vi "Cannon Auto.vi"(1 "Cannon Info In":T2) -> (0 "Cannon Info Out":T2)   [LabVIEW 2013]
uses:
  <vilib>/Rock Robotics/WPI/Solenoid/WPI_SolenoidValue.ctl
panel:
  # "Togle"
  # "Togle"
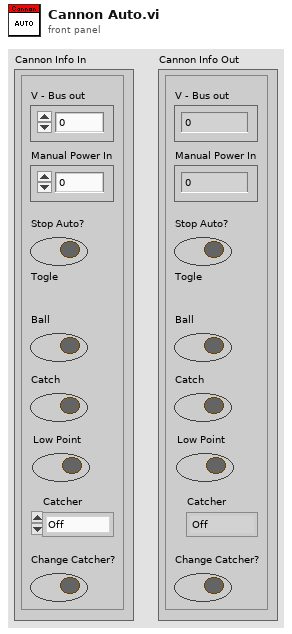
[diagram p1: front panel]
types:
  T1 = typedef "WPI_SolenoidValue.ctl" = enum16{"Off", "On", "Forward", "Reverse"}
  T2 = cluster{"V - Bus out":dbl, "Manual Power In":dbl, "Stop Auto?":bool, "Ball":bool, "Catch":bool, "Low Point":bool, "Catcher":T1, "Change Catcher?":bool}
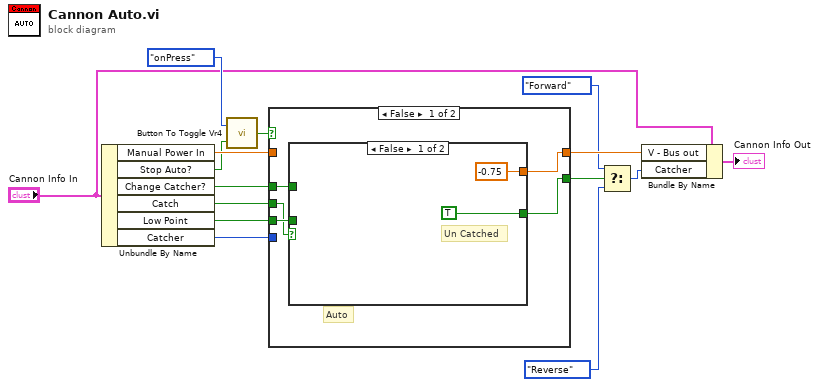
[diagram p0: block diagram]
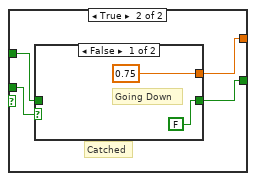
[diagram p2: hidden frame]
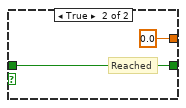
[diagram p3: hidden frame]
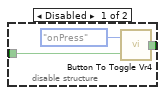
[diagram p5: hidden frame]
diagram:
  n1 = Unbundle By Name("Cannon Info In") -> ("Manual Power In"=w11:dbl, "Stop Auto?"=w1:bool, "Change Catcher?"=w3:bool, "Catch"=w13:bool, "Low Point"=w12:bool, "Catcher"=w2:T1)
  n2 = call "Button To Toggle Vr4.vi"("InValue"=w1, "Action"=enum16{"onPress", "onRelease", "Both"}."onPress") -> ("Result"=w14:bool)
  n3 = case shown="False" w14 {
    tunnel: w13 -> [w17 _]
    tunnel: w12 -> [w20 _]
    tunnel: w11 -> [_ w33]
    tunnel: w3 -> [w16 w32]
    tunnel: [w18 w33] -> w8
    tunnel: [w19 w31] -> w7
    tunnel: w2 -> [_ _]
    frame False {
      # "Auto"
      n4 = case shown="False" w17 {
        tunnel: w20 -> [_ w26]
        tunnel: [TRUE w24] -> w19
        tunnel: [-0.75 w25] -> w18
        tunnel: w16 -> [_ w23]
        frame False {
          # "Un Catched"
        }
        frame True {
          # "Catched"
          n5 = case shown="False" w26 {
            tunnel: [0.75 0.0] -> w25
            tunnel: [FALSE w29] -> w24
            tunnel: w23 -> [_ w29]
            frame False {
              # "Going Down"
            }
            frame True {
              # "Reached"
            }
          }
        }
      }
    }
    frame True {
      n6 = disable-structure shown="Enabled" {
        disable-tunnel: w32 -> [w35 w37]
        disable-tunnel: [w34 w37] -> w31
        frame Disabled {
          n7 = call "Button To Toggle Vr4.vi"("InValue"=w35, "Action"=enum16{"onPress", "onRelease", "Both"}."onPress") -> ("Result"=w34:bool)
        }
        frame Enabled {
        }
      }
    }
  }
  n8 = Select(t=WPI_SolenoidValue."Forward" ("Catcher"), s=w7, f=WPI_SolenoidValue."Reverse" ("Catcher")) -> (s? t:f=w4:T1)
  n9 = Bundle By Name(cluster="Cannon Info In", "V - Bus out"=w8, "Catcher"=w4) -> (→"Cannon Info Out":T2)
